vi "Test Configure Audio Device Duplicate.vi"(8 "error in (no error)":errorcluster) -> (0 "error out":errorcluster, 3 "Pass?":bool)   [LabVIEW 2020]
uses:
  G-Audio/G-Audio.lvlib
  <vilib>/Utility/error.llb/Error Cluster From Error Code.vi
  <vilib>/ErrorRing/Error Ring.xnode
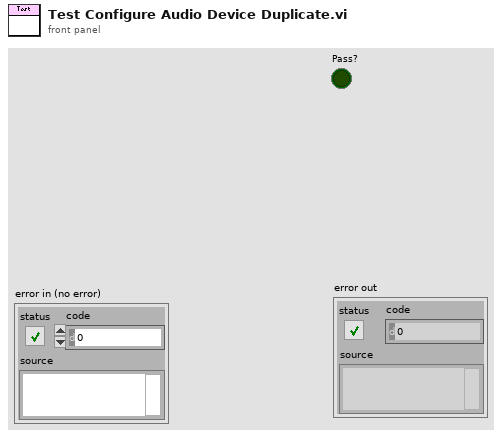
[diagram p1: front panel]
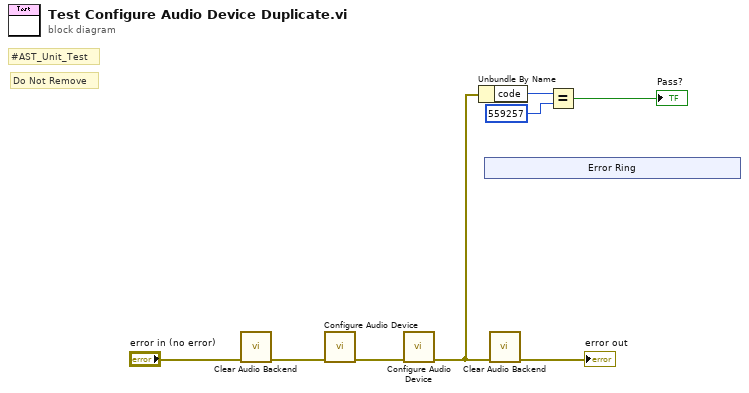
[diagram p0: block diagram]
diagram:
  # "Do Not Remove"
  # "#AST_Unit_Test"
  n1 = call "Clear Audio Backend.vi"("error in (no error)"="error in (no error)") -> ("error out"=w7:errorcluster)  [unwired: 10 in]
  n2 = call "Configure Audio Device.vi"("error in (no error)"=w7) -> ("error out"=w6:errorcluster)  [unwired: 7 in, 3 out]
  n3 = call "Configure Audio Device.vi"("error in (no error)"=w6) -> ("error out"=w2:errorcluster)  [unwired: 7 in, 3 out]
  n4 = Unbundle By Name(w2) -> ("code"=w5:i32)
  n5 = xnode "Error Ring"() -> ()  [unwired: 1 out]
  n6 = call "Clear Audio Backend.vi"("error in (no error)"=w2) -> ("error out"=→"error out":errorcluster)  [unwired: 10 in]
  n7 = Equal?(x=w5, y=559257) -> (x = y?=→"Pass?":bool)
